vi "ForecastNightDay.vi"(8 "Fehler (Eingang, kein Fehler)":errorcluster, 10 "DataFlowIN (Eingang)":T1, 11 "TableName":string) -> (0 "Fehler (Ausgang)":errorcluster, 1 "Daytime":i32, 2 "Night(22-6)?":bool, 3 "DataFlowIN (Ausgang)":T1)   [LabVIEW 2017]
uses:
  classes/DataCollector.lvclass
  classes/DataHandler.lvclass
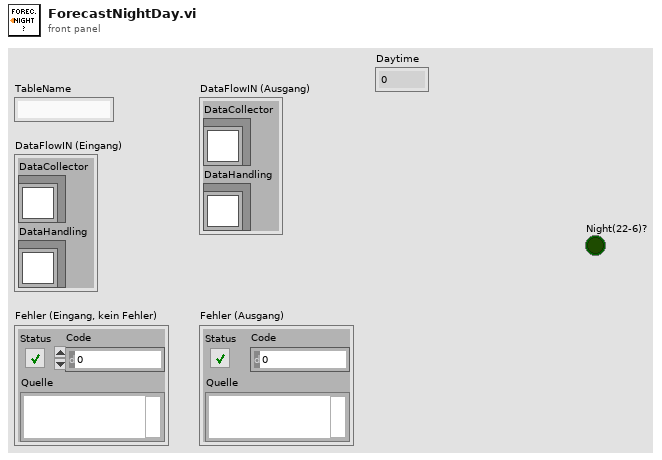
[diagram p1: front panel]
types:
  T1 = cluster{"DataCollector":refnum<class "DataCollector.lvclass">, "DataHandling":refnum<class "DataHandler.lvclass">}
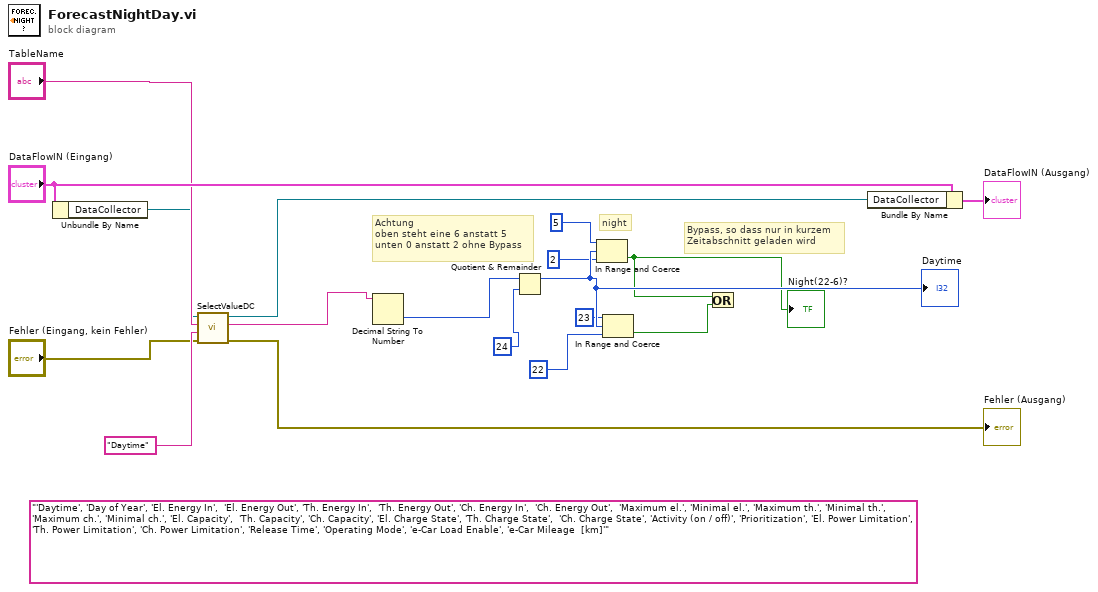
[diagram p0: block diagram]
diagram:
  (unwired) "'Daytime', 'Day of Year', 'El. Energy In',  'El. Energy Out', 'Th. Energy In',  'Th. Energy Out', 'Ch. Energy In',  'Ch. Energy Out',  'Maximum el.', 'Minimal el.', 'Maximum th.', 'Minimal th.',  'Maximum ch.', 'Minimal ch.', 'El. Capacity',  'Th. Capacity', 'Ch. Capacity', 'El. Charge State', 'Th. Charge State',  'Ch. Charge State', 'Activity (on / off)', 'Prioritization', 'El. Power Limitation',  'Th. Power Limitation', 'Ch. Power Limitation', 'Release Time', 'Operating Mode', 'e-Car Load Enable', 'e-Car Mileage  [km]'" ("string")
  # "Achtung\noben steht eine 6 anstatt 5\nunten 0 anstatt 2 ohne Bypass"
  # "Bypass, so dass nur in kurzem\nZeitabschnitt geladen wird"
  # "night"
  n1 = Unbundle By Name("DataFlowIN (Eingang)") -> ("DataCollector"=w11:refnum<class "DataCollector.lvclass">)
  n2 = call-dynamic "SelectValueDC.vi"("error in (no error)"="Fehler (Eingang, kein Fehler)", "Table Row Name"="Daytime", "Unique Object Identifier"="TableName", "DataCollector in"=w11) -> ("error out"=→"Fehler (Ausgang)":errorcluster, "Value"=w10:string, "DataCollector out"=w18:refnum<class "DataCollector.lvclass">)  [unwired: 5 in]
  n3 = Decimal String To Number(string=w10) -> (number=w2:i32)  [unwired: 2 in, 1 out]
  n4 = Quotient & Remainder(x=w2, y=24) -> (x-y*floor(x/y)=w9:i32)  [unwired: 1 out]
  "Daytime" <- w9
  n5 = In Range and Coerce(upper limit=5 ("Obergrenze"), x=w9, lower limit=u32 2 ("Untergrenze")) -> (In Range?=w1:bool)  [unwired: 1 out]
  "Night(22-6)?" <- w1
  n6 = In Range and Coerce(upper limit=23 ("Obergrenze"), x=w9, lower limit=22 ("Obergrenze")) -> (In Range?=w5:bool)  [unwired: 1 out]
  n7 = Or(x=w1, y=w5) -> ()  [unwired: 1 out]
  n8 = Bundle By Name(cluster="DataFlowIN (Eingang)", "DataCollector"=w18) -> (→"DataFlowIN (Ausgang)":T1)
